vi "Read Min Max Waveform.vi"(8 "error in (no error)":errorcluster {"code" format="%.0x"}, 10 "Channel Name (\"Channel 1\")":string(combo)="CHAN1", 11 "VISA Resource Name":refnum<visa-resource-name>) -> (0 "error out":errorcluster {"code" format="%.0x"}, 1 "x increment":dbl caption="x Increment" format="%^.2e", 2 "initial x":dbl caption="Initial x" format="%^.2e", 3 "VISA Resource Name Out":refnum<visa-resource-name>, 4 "Max waveform array":dbl[](array[numeric]) caption="Max Waveform Array" format="%.2f", 5 "actual points":u32 caption="Actual Points", 6 "Min waveform array":dbl[](array[numeric]) caption="Min Waveform Array" format="%.2f")   [LabVIEW 2011, in "Agilent 546XX Series.lvlib"]
doc: "This VI initiates an acquisition on the channels that you enable with the ag546xx Configure Channel VI. It then waits for the acquisition to complete, and returns the min/max waveforms for the channel you specify. You call the ag546xx Fetch Min Max Waveform VI to obtain the min/max waveforms for each of the remaining enabled channels without initiating another acquisition.\n\nUse this VI to read waveforms when you set the acquisition type to Peak Detect.\n\nNotes:\n\n(1) After this VI executes, each element in the Min Waveform Array and Max Waveform Array is either a voltage or a value indicating that the oscilloscope could not sample a voltage."
uses:
  Agilent 546XX Series.lvlib
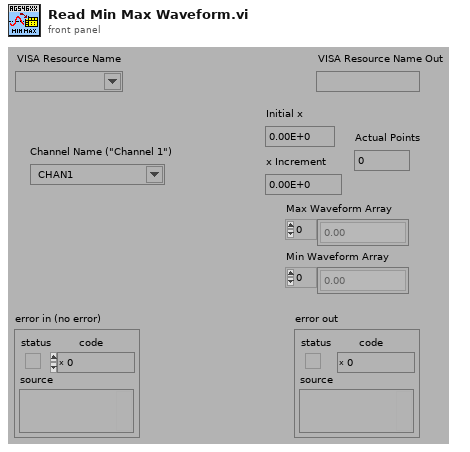
[diagram p1: front panel]
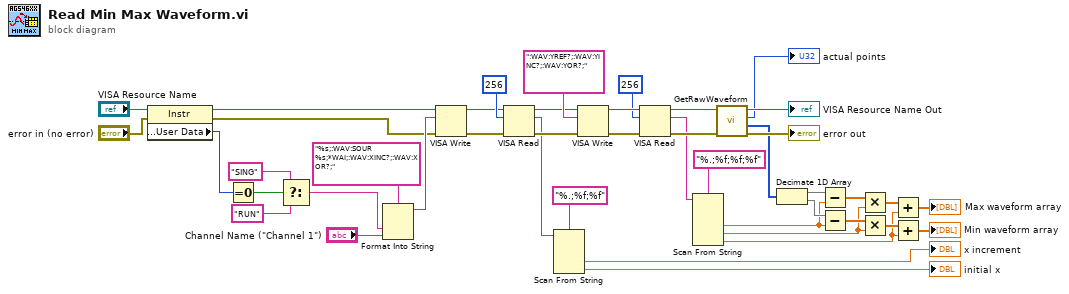
[diagram p0: block diagram]
diagram:
  n1 = property class="Instr"(reference="VISA Resource Name", error in="error in (no error)") -> (reference out=w27:refnum<visa-resource-name>, error out=w26:errorcluster, "General Settings:User Data"=w24:u32)
  n2 = Equal To 0?(x=w24) -> (x = 0?=w25:bool)
  n3 = Select(t="SING", s=w25, f="RUN") -> (s? t:f=w20:string)
  n4 = Format Into String(format string="%s;:WAV:SOUR %s;*WAI;:WAV:XINC?;:WAV:XOR?;", w20, "Channel Name (\"Channel 1\")") -> (resulting string=w43:string)  [unwired: 2 in, 1 out]
  n5 = VISA Write(VISA resource name=w27, write buffer=w43, error in (no error)=w26) -> (VISA resource name out=w6:refnum<visa-resource-name>, error out=w8:errorcluster)  [unwired: 1 out]
  n6 = VISA Read(VISA resource name=w6, byte count=u32 256, error in (no error)=w8) -> (VISA resource name out=w5:refnum<visa-resource-name>, read buffer=w3:string, error out=w7:errorcluster)  [unwired: 1 out]
  n7 = Scan From String(format string="%.;%f;%f", input string=w3) -> (output 1=→"x increment":dbl, output 2=→"initial x":dbl)  [unwired: 4 in, 3 out]
  n8 = VISA Write(VISA resource name=w5, write buffer=":WAV:YREF?;:WAV:YINC?;:WAV:YOR?;", error in (no error)=w7) -> (VISA resource name out=w42:refnum<visa-resource-name>, error out=w41:errorcluster)  [unwired: 1 out]
  n9 = VISA Read(VISA resource name=w42, byte count=u32 256, error in (no error)=w41) -> (VISA resource name out=w40:refnum<visa-resource-name>, read buffer=w34:string, error out=w39:errorcluster)  [unwired: 1 out]
  n10 = Scan From String(format string="%.;%f;%f;%f", input string=w34) -> (output 1=w12:dbl, output 2=w14:dbl, output 3=w13:dbl)  [unwired: 5 in, 3 out]
  n11 = call "GetRawWaveform.vi"("error in"=w39, "VISA Resource Name"=w40) -> ("error out"=→"error out":errorcluster, "Waveform Array"=w19:u32[], "Number of Points"=→"actual points":u32, "VISA Resource Name Out"=→"VISA Resource Name Out":refnum<visa-resource-name>)  [unwired: 5 in, 1 out]
  n12 = Decimate 1D Array(w19) -> (w15:u32[], w18:u32[])
  n13 = Subtract(x=w15, y=w12) -> (x-y=w16:dbl[])
  n14 = Subtract(x=w18, y=w12) -> (x-y=w32:dbl[])
  n15 = Multiply(x=w16, y=w14) -> (x*y=w17:dbl[])
  n16 = Multiply(x=w32, y=w14) -> (x*y=w31:dbl[])
  n17 = Add(x=w17, y=w13) -> (x+y=→"Max waveform array":dbl[])
  n18 = Add(x=w31, y=w13) -> (x+y=→"Min waveform array":dbl[])
